vi "Show Error Dialog.vi"(8 "error in (no error)":errorcluster, 10 "Error Message Data":T1, 11 "Error Handler In":refnum<class "Error Handler.lvclass">) -> (0 "error out":errorcluster, 3 "Error Handler Out":refnum<class "Error Handler.lvclass">)   [LabVIEW 2020, in "Error Handler.lvclass"]
uses:
  Error Handler.lvclass
  Public/TypeDefs/Error Message Data.ctl
  Error Handler.lvclass/Error Handler.ctl
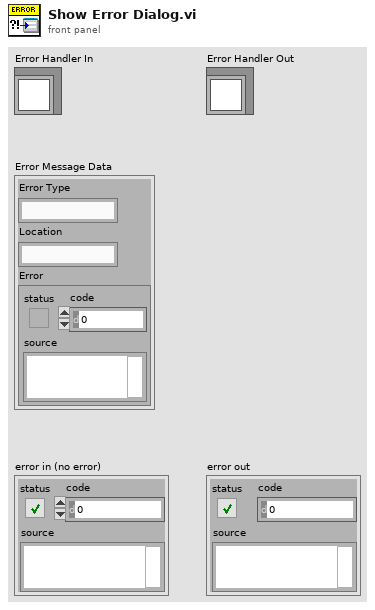
[diagram p1: front panel]
types:
  T1 = typedef "Error Handler.lvclass/Error Message Data.ctl" = cluster{"Error Type":string, "Location":string, "Error":errorcluster}
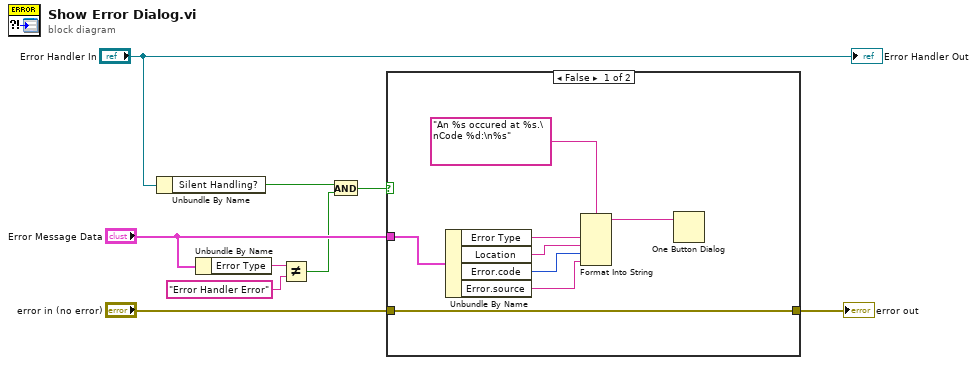
[diagram p0: block diagram]
diagram:
  n1 = Unbundle By Name("Error Handler In") -> ("Silent Handling?"=w8:bool)
  n2 = Unbundle By Name("Error Message Data") -> ("Error Type"=w4:string)
  n3 = Not Equal?(x=w4, y="Error Handler Error" ("Error Type")) -> (x != y?=w1:bool)
  n4 = And(x=w8, y=w1) -> (x .and. y?=w2:bool)
  n5 = case shown="False" w2 {
    tunnel: "Error Message Data" -> [w16 _]
    tunnel: "error in (no error)" -> [w17 w18]
    tunnel: [w17 w18] -> w6
    frame False {
      n6 = Unbundle By Name(w16) -> ("Error Type"=w14:string, "Location"=w13:string, "Error.code"=w12:i32, "Error.source"=w11:string)
      n7 = Format Into String(format string="An %s occured at %s.\nCode %d:\n%s", w14, w13, w12, w11) -> (resulting string=w10:string)  [unwired: 2 in, 1 out]
      n8 = One Button Dialog(message=w10) -> ()  [unwired: 1 in, 1 out]
    }
    frame True {
    }
  }
  "error out" <- w6
  "Error Handler Out" <- "Error Handler In"
